vi "Test REST Credentials.vi"(8 "error in (no error)":errorcluster, 10 "API Key":string, 11 "REST URL":string) -> (0 "error out":errorcluster)   [LabVIEW 2024, in "Sift TDMS Uploader.lvlib" / "Sift TDMS Uploader.lvclass"]
doc: "Calls Sift Ping endpoint to validate API key and REST URL."
uses:
  Sift TDMS Uploader.lvclass
  <vilib>/regexp/Match Regular Expression.xnode
  <vilib>/httpClient/LabVIEWHTTPClient.lvlib
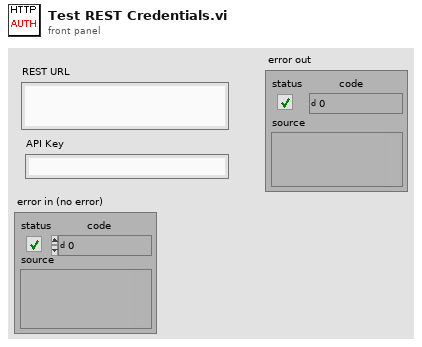
[diagram p1: front panel]
types:
  T1 = typedef "LabVIEWHTTPClient.lvlib/ClientHandle.ctl" = refnum<k1>
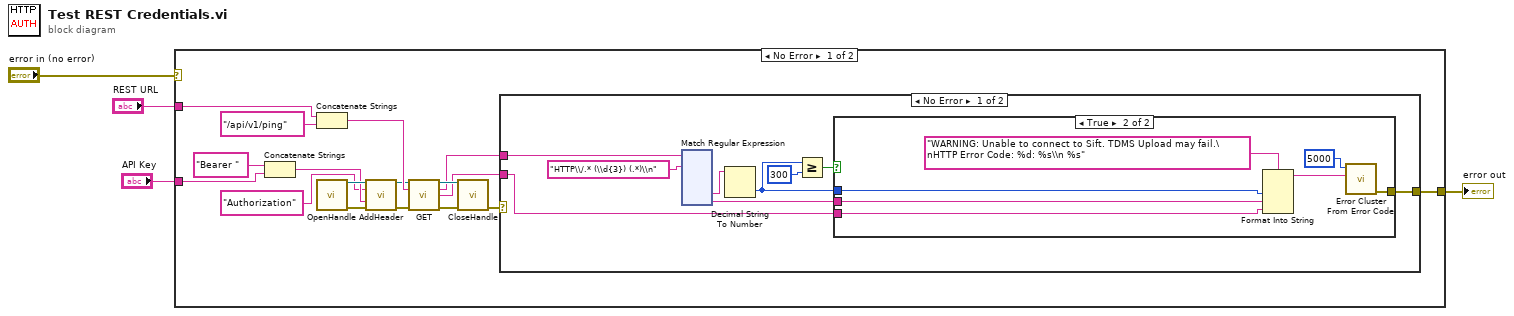
[diagram p0: block diagram]
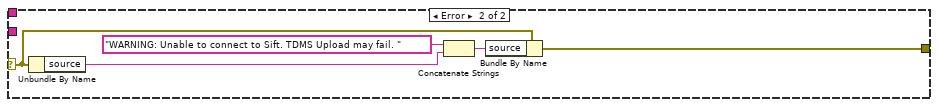
[diagram p3: hidden frame]
diagram:
  n1 = case shown="No Error" "error in (no error)" {
    tunnel: "REST URL" -> [w21 _]
    tunnel: "API Key" -> [w15 _]
    tunnel: [w6 _] -> w1
    frame No Error {
      n2 = Concatenate Strings("Bearer ", w15) -> (w14:string)
      n3 = Concatenate Strings(w21, "/api/v1/ping") -> (w19:string)
      n4 = call <vilib>:"OpenHandle.vi"() -> ("client handle out"=w18:T1, "error out"=w10:errorcluster)  [unwired: 14 in]
      n5 = call <vilib>:"AddHeader.vi"("client handle"=w18, "header"="Authorization", "value"=w14, "error in (no error)"=w10) -> ("client handle out"=w17:T1, "error out"=w11:errorcluster)  [unwired: 10 in]
      n6 = call <vilib>:"GET.vi"("client handle"=w17, "url"=w19, "error in (no error)"=w11) -> ("client handle out"=w12:T1, "headers"=w8:string, "body"=w7:string, "error out"=w9:errorcluster)  [unwired: 9 in]
      n7 = call <vilib>:"CloseHandle.vi"("client handle"=w12, "error in (no error)"=w9) -> ("error out"=w5:errorcluster)  [unwired: 13 in]
      n8 = case shown="No Error" w5 {
        selector: w5 -> [_ w162]
        tunnel: w8 -> [w28 _]
        tunnel: w7 -> [w23 _]
        tunnel: [w22 w158] -> w6
        frame No Error {
          n9 = xnode "Match Regular Expression"("input string"=w28, "regular expression"="HTTP\\/.* (\\d{3}) (.*)\\n") -> ("submatch 1"=w25:string, "submatch 2"=w26:string)  [unwired: 4 in, 5 out]
          n10 = Decimal String To Number(string=w25) -> (number=w24:i32)  [unwired: 2 in, 1 out]
          n11 = Greater Or Equal?(x=w24, y=300) -> (x >= y?=w29:bool)
          n12 = case shown="True" w29 {
            tunnel: [_ w157] -> w22
            tunnel: w26 -> [_ w152]
            tunnel: w24 -> [_ w154]
            tunnel: w23 -> [_ w153]
            frame False {
            }
            frame True {
              n13 = Format Into String(format string="WARNING: Unable to connect to Sift. TDMS Upload may fail.\nHTTP Error Code: %d: %s\\n %s", w154, w152, w153) -> (resulting string=w151:string)  [unwired: 2 in, 1 out]
              n14 = call <vilib>:"Error Cluster From Error Code.vi"("error message (\"\")"=w151, "error code (0)"=5000) -> ("error out"=w157:errorcluster)  [unwired: 7 in]
            }
          }
        }
        frame Error {
          n15 = Unbundle By Name(w162) -> ("source"=w160:string)
          n16 = Concatenate Strings("WARNING: Unable to connect to Sift. TDMS Upload may fail. ", w160) -> (w159:string)
          n17 = Bundle By Name(cluster=w162, "source"=w159) -> (w158:errorcluster)
        }
      }
    }
    frame Error {
    }
  }
  "error out" <- w1
